vi "CfgFile Set Desc Menu.vi"(8 "error in (no error)":errorcluster, 10 "Menu":T1, 11 "LF2R IDE in":refnum<class "LF2R IDE.lvclass">) -> (0 "error out":errorcluster, 3 "LF2R IDE out":refnum<class "LF2R IDE.lvclass">)   [LabVIEW 2018, in "LF2R IDE.lvlib" / "LF2R IDE.lvclass"]
uses:
  LF2R IDE.lvclass
  Const UI Desc Menu.ctl
  Const UI Desc Property.ctl
  Menu Item.ctl
  LF2R IDE.lvclass/LF2R IDE.ctl
  <userlib>/_MGI/Menu Building/MenuItem/MGI_MenuItem.lvclass
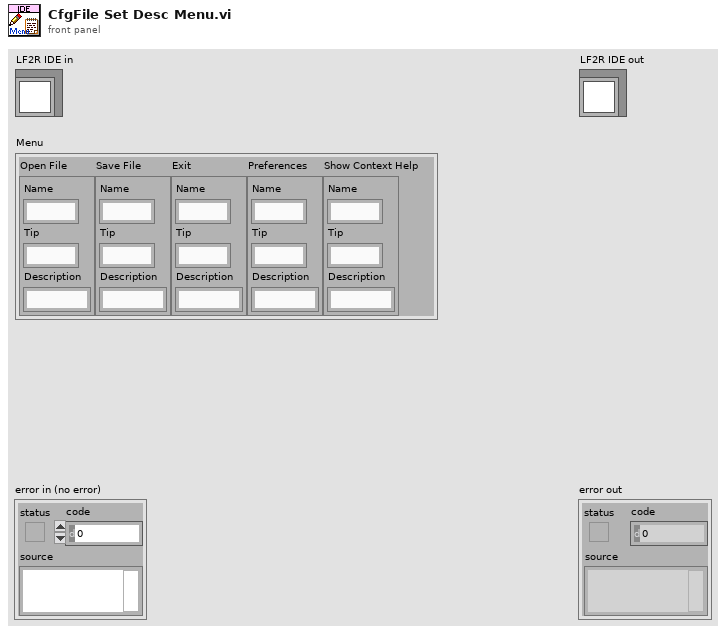
[diagram p1: front panel]
types:
  T1 = typedef "LF2R IDE.lvlib/LF2R IDE.lvclass/Const UI Desc Menu.ctl" = cluster{"Open File":T2, "Save File":T2, "Exit":T2, "Preferences":T2, "Show Context Help":T2}
  T2 = typedef "LF2R IDE.lvlib/LF2R IDE.lvclass/Const UI Desc Property.ctl" = cluster{"Name":string, "Tip":string, "Description":string}
  T3 = typedef "LF2R IDE.lvlib/LF2R IDE.lvclass/Menu Item.ctl" = enum16{"Invalid Item", "Open File", "Save File", "Exit", "Preferences", "Show Context Help"}
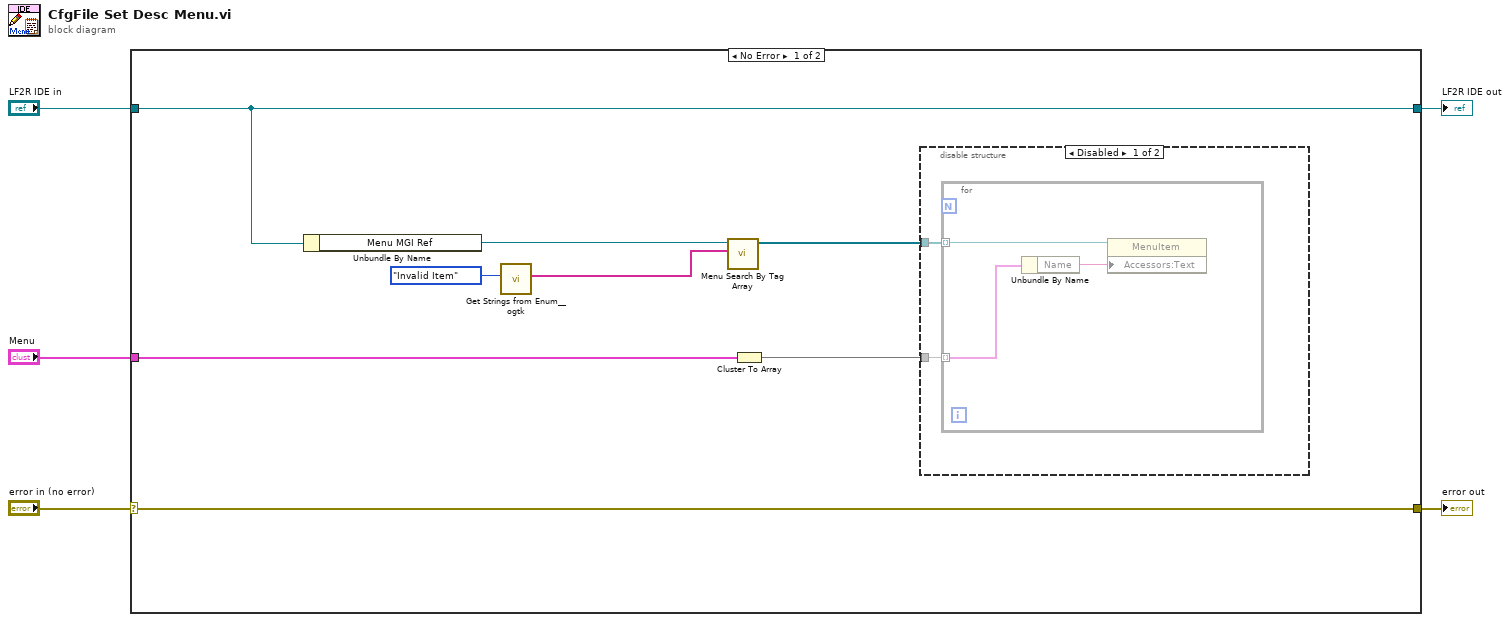
[diagram p0: block diagram]
diagram:
  n1 = case shown="No Error" "error in (no error)" {
    selector: "error in (no error)" -> [w11 w20]
    tunnel: [w11 w20] -> w4
    tunnel: [w13 w19] -> w2
    tunnel: "LF2R IDE in" -> [w13 w19]
    tunnel: "Menu" -> [w7 _]
    frame No Error {
      n2 = Unbundle By Name(w13) -> ("Menu MGI Ref"=w12:refnum<class "MGI_VI.lvclass">)
      n3 = call <userlib>:"Get Strings from Enum__ogtk.vi"("Enum"=Menu_Item."Invalid Item" ("Menu Item")) -> ("Enum Strings"=w9:string[])  [unwired: 7 in, 3 out]
      n4 = call "Menu Search By Tag Array.vi"("Tag Array"=w9, "Menu MGI Ref"=w12) -> ("Menu Item Array"=w8:refnum<data-value>[])  [unwired: 7 in, 2 out]
      n5 = Cluster To Array(cluster=w7) -> (array=w6:T2[])
      n6 = disable-structure shown="Disabled" {
        disable-tunnel: w8 -> [w15 _]
        disable-tunnel: w6 -> [w14 _]
        frame Disabled {
          n7 = for {
            tunnel: w15 -> [w18] mode=indexing
            tunnel: w14 -> [w17] mode=indexing
            n8 = Unbundle By Name(w17) -> ("Name"=w16:string)
            n9 = property class="MenuItem"(reference=w18, "Accessors:Text"=w16) -> ()  [unwired: 1 in, 2 out]
          }
        }
        frame Enabled {
        }
      }
    }
    frame Error {
    }
  }
  "error out" <- w4
  "LF2R IDE out" <- w2
